vi "Omega Temp Server.vi"() -> ()   [LabVIEW 2019]
doc: "This VI reads a single reading from an Omega CNi32 temperature controller. The stop boolean is always false. If no reading is obtained a single zero is returned. Adapted from code by Scott Hannahs.\nJonathan Billings, NHMFL-FSU, Jan 2008"
panel:
  in  "Submit":bool
  in  "Set Point #2":dbl
  in  "Set Point #1":dbl
  out "CNi32 Current Reading":dbl(slide) scale=70.0..100.0
  in  "Halt":bool
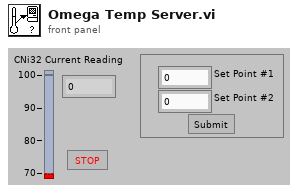
[diagram p1: front panel]
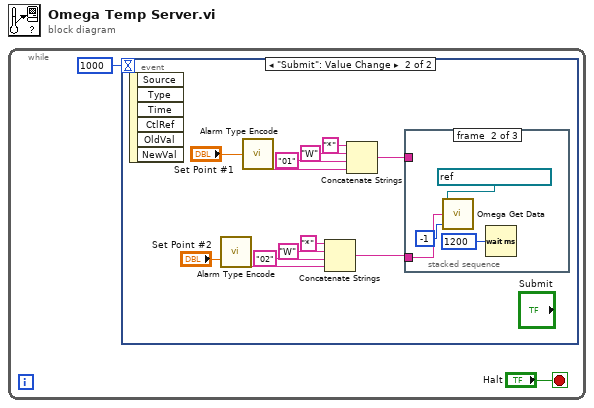
[diagram p0: block diagram]
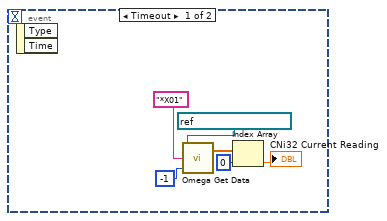
[diagram p2: hidden frame]
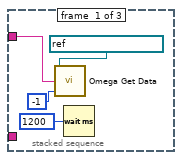
[diagram p3: hidden frame]
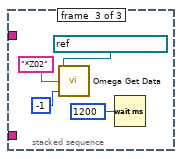
[diagram p4: hidden frame]
diagram:
  n1 = while {
    stop <- "Halt" stop-if-true
    n2 = event shown="[1] \"Submit\": Value Change" {
      selector: _ -> [_ _]
      dyn-events: _ -> [_ _]
      timeout: 1000 -> [_ _]
      event Timeout {
        n3 = event-data() -> ()  [unwired: 1 in, 2 out]
        n4 = call "Omega Get Data.vi"("Point #"=-1, "Command String"="*X01", "GPIB Address"=refnum<visa-resource-name> "GPIB0::2::INSTR") -> ("Measurement"=w8:dbl[])  [unwired: 1 out]
        n5 = Index Array(array=w8, index=0) -> (element=→"CNi32 Current Reading":dbl)
      }
      event "Submit": Value Change {
        n6 = event-data() -> ()  [unwired: 1 in, 6 out]
        n7 = call "Alarm Type Encode.vi"("Input"="Set Point #2") -> ("resulting string"=w16:string)
        n8 = call "Alarm Type Encode.vi"("Input"="Set Point #1") -> ("resulting string"=w9:string)
        n9 = Concatenate Strings("*" ("string"), "W" ("Command Class"), "02" ("Command Suffix"), w16) -> (w19:string)
        n10 = Concatenate Strings("*" ("string"), "W" ("Command Class"), "01" ("Command Suffix"), w9) -> (w10:string)
        n11 = stacked-sequence {
          tunnel: w10 -> [w22 _ _]
          tunnel: w19 -> [_ w26 _]
          frame #0 {
            n12 = call "Omega Get Data.vi"("Point #"=-1, "Command String"=w22, "GPIB Address"=refnum<visa-resource-name> "GPIB0::2::INSTR") -> ()  [unwired: 2 out]
            n13 = Wait (ms)(milliseconds to wait=u32 1200) -> ()  [unwired: 1 out]
          }
          frame #1 {
            n14 = call "Omega Get Data.vi"("Point #"=-1, "Command String"=w26, "GPIB Address"=refnum<visa-resource-name> "GPIB0::2::INSTR") -> ()  [unwired: 2 out]
            n15 = Wait (ms)(milliseconds to wait=u32 1200) -> ()  [unwired: 1 out]
          }
          frame #2 {
            n16 = call "Omega Get Data.vi"("Point #"=-1, "Command String"="*Z02", "GPIB Address"=refnum<visa-resource-name> "GPIB0::2::INSTR") -> ()  [unwired: 2 out]
            n17 = Wait (ms)(milliseconds to wait=u32 1200) -> ()  [unwired: 1 out]
          }
        }
      }
    }
  }
